vi "enum wrap.vi"() -> ()   [LabVIEW 2013]
panel:
  out "Enum":enum16{"0", "1", "2", "3", "4"}(ring)
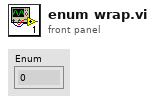
[diagram p1: front panel]
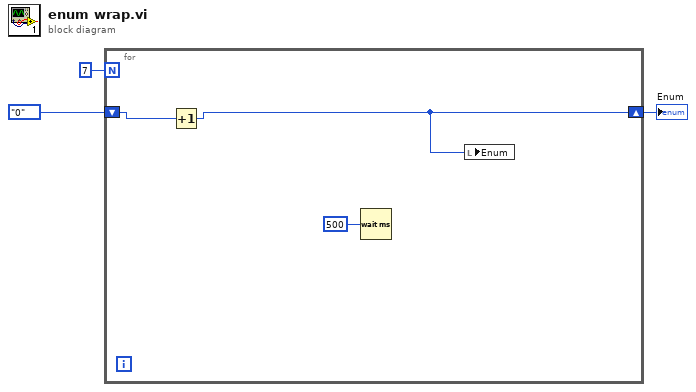
[diagram p0: block diagram]
diagram:
  n1 = for {
    N: 7 -> [_]
    shift-right: [w4] -> w2
    shift-left: enum16{"0", "1", "2", "3", "4"}."0" -> [w6]
    n2 = Increment(x=w6) -> (x+1=w4:enum16{"0", "1", "2", "3", "4"})
    n3 = Wait (ms)(milliseconds to wait=u32 500) -> ()  [unwired: 1 out]
    n4 = local write "Enum"(w4) -> ()
  }
  "Enum" <- w2
